vi "AOTFInit.vi"(1 "error in (no error)":errorcluster) -> (0 "error out":errorcluster)   [LabVIEW 2009]
uses:
  AOTFSettings.ctt
  <vilib>/Utility/config.llb/NI_LVConfig.lvlib
panel:
  out "AOTF Setting":T1={"Laser 1 Output Channel"="5", "AOTF  1 Output Voltage"=2.0, "Laser 2 Output Channel"="6", "AOTF  2 Output Voltage"=5.0, "Laser 3 Output Channel"="1", "AOTF  3 Output Voltage"=0.0, "Pixel per Cycle"=0, "Time per Cycle  / ms"=10.0, "Laser 4 Output Channel"="1", "AOTF  4 Output Voltage"=0.0} {"AOTF  4 Output Voltage" format="%.2f"; "Time per Cycle  / ms" format="%#.3f"; "AOTF  3 Output Voltage" min=0.0 max=10.0 format="%.2f"; "AOTF  2 Output Voltage" min=0.0 max=10.0 format="%.2f"; "AOTF  1 Output Voltage" min=0.0 max=10.0 format="%.2f"}
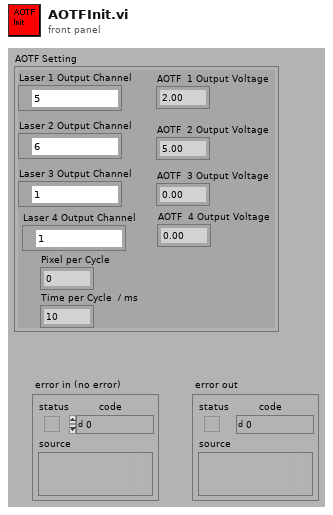
[diagram p1: front panel]
types:
  T1 = typedef "AOTFSettings.ctt" = cluster{"Laser 1 Output Channel":tag, "AOTF  1 Output Voltage":dbl, "Laser 2 Output Channel":tag, "AOTF  2 Output Voltage":dbl, "Laser 3 Output Channel":tag, "AOTF  3 Output Voltage":dbl, "Pixel per Cycle":u16, "Time per Cycle  / ms":dbl, "Laser 4 Output Channel":tag, "AOTF  4 Output Voltage":dbl}
  T2 = typedef "NI_LVConfig.lvlib/Config Data RefNum.ctl" = refnum<k1>
  T3 = cluster{"Laser 1 Output Channel":tag, "AOTF  1 Output Voltage":dbl, "Laser 2 Output Channel":tag, "AOTF  2 Output Voltage":dbl, "Laser 3 Output Channel":tag, "AOTF  3 Output Voltage":dbl, "Pixel per Cycle":u16, "Time per Cycle  / ms":dbl, "Laser 4 Output Channel":tag, "AOTF  4 Output Voltage":dbl}
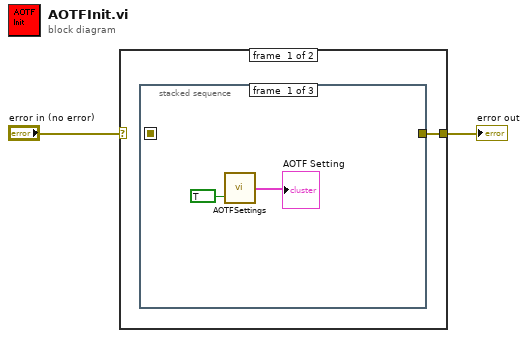
[diagram p0: block diagram]
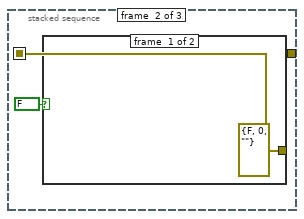
[diagram p2: hidden frame]
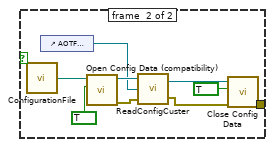
[diagram p3: hidden frame]
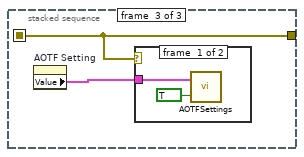
[diagram p4: hidden frame]
diagram:
  n1 = case shown="No Error" "error in (no error)" {
    selector: "error in (no error)" -> [_ w22]
    tunnel: [w3 w22] -> w1
    frame #0 {
      n2 = stacked-sequence {
        seq-local: [_ w7 _] -> [_ _ w18]
        tunnel: [_ _ w18] -> w3
        frame #0 {
          n3 = call "AOTFSettings.vi"("Get/Set"=TRUE) -> ("AOTF Setting (Output)"=→"AOTF Setting":T1)  [unwired: 1 in]
        }
        frame #1 {
          n4 = case shown="True" FALSE {
            tunnel: [errorcluster {"status"=FALSE, "code"=0, "source"=""} ("error out") w13] -> w7
            frame #0 {
            }
            frame #1 {
              n5 = call "ConfigurationFile.vi"() -> ("Configuration File (output)"=w12:path)  [unwired: 2 in]
              n6 = control-ref of="AOTF Setting"() -> (w9:refnum<vi>)
              n7 = call <vilib>:"Open Config Data (compatibility).vi"("create file if necessary (T)"=TRUE ("create file if necessary? (T)"), "configuration file path"=w12) -> ("error out"=w15:errorcluster, "refnum"=w16:T2)  [unwired: 7 in, 1 out]
              n8 = call "ReadConfigCuster.vi"("error in (no error)"=w15, "Ctrl Reference"=w9, "ConfigFile (input)"=w16) -> ("error out"=w10:errorcluster, "ConfigFile (output)"=w11:T2)
              n9 = call "Close Config Data.vi"("error in (no error)"=w10, "write configuration file? (T)"=TRUE ("write configuration file? (F)"), "refnum"=w11) -> ("error out"=w13:errorcluster)  [unwired: 8 in]
            }
          }
        }
        frame #2 {
          n10 = property on="AOTF Setting" class="Cluster (strikt)"() -> ("Value"=w19:T3)  [unwired: 2 in, 2 out]
          n11 = case shown="No Error" w18 {
            tunnel: w19 -> [w20 _]
            frame #0 {
              n12 = call "AOTFSettings.vi"("Get/Set"=TRUE ("Set"), "AOTF Setting (Input)"=w20) -> ()  [unwired: 1 out]
            }
            frame #1 {
            }
          }
        }
      }
    }
    frame #1 {
    }
  }
  "error out" <- w1
